vi "FL Sigmoid COA Single Side.vi"(0 "weight":dbl, 5 "Implication":T1 items=["Minimum", "Product"], 7 "x0":dbl=-5.0, 9 "x1":dbl=5.0, 11 "A":dbl=1.0) -> (4 "xlh":dbl, 6 "area":dbl, 8 "coa_x":dbl, 10 "x_l":dbl, 15 "x_r":dbl)   [LabVIEW 2017, in "NI_Fuzzy_Logic_API.lvlib"]
uses:
  <vilib>/addons/Fuzzy Logic/NI_Fuzzy_Logic_API.lvlib
  <vilib>/addons/Fuzzy Logic/TypeDefs/FL Consequent Implication.ctl
  <vilib>/gmath/NI_Gmath.lvlib
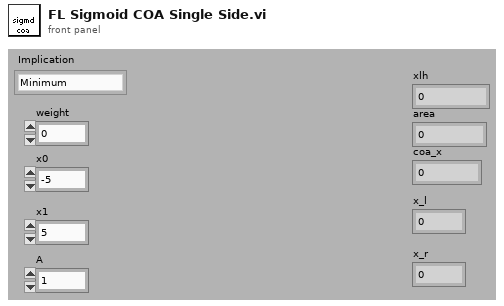
[diagram p1: front panel]
types:
  T1 = typedef "NI_Fuzzy_Logic_API.lvlib/FL Consequent Implication.ctl" = u16
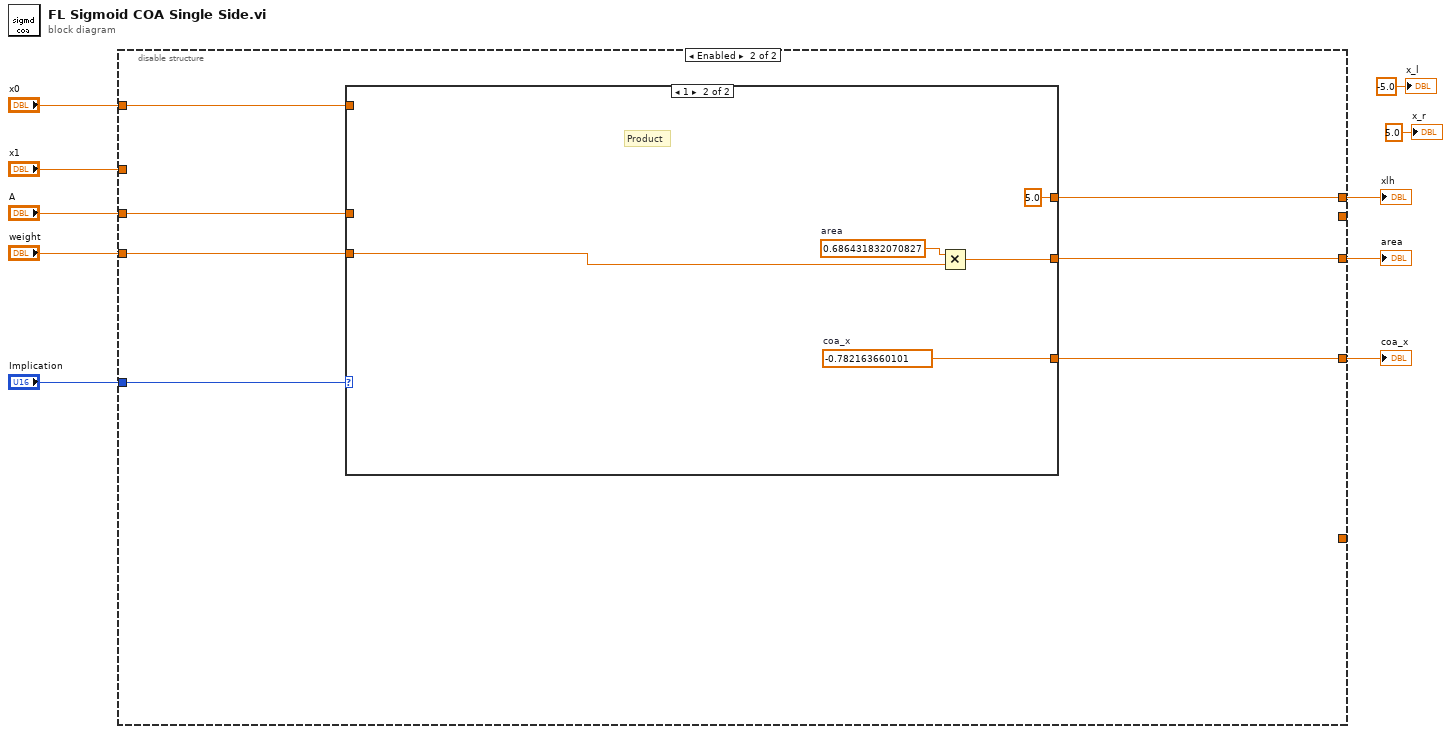
[diagram p0: block diagram]
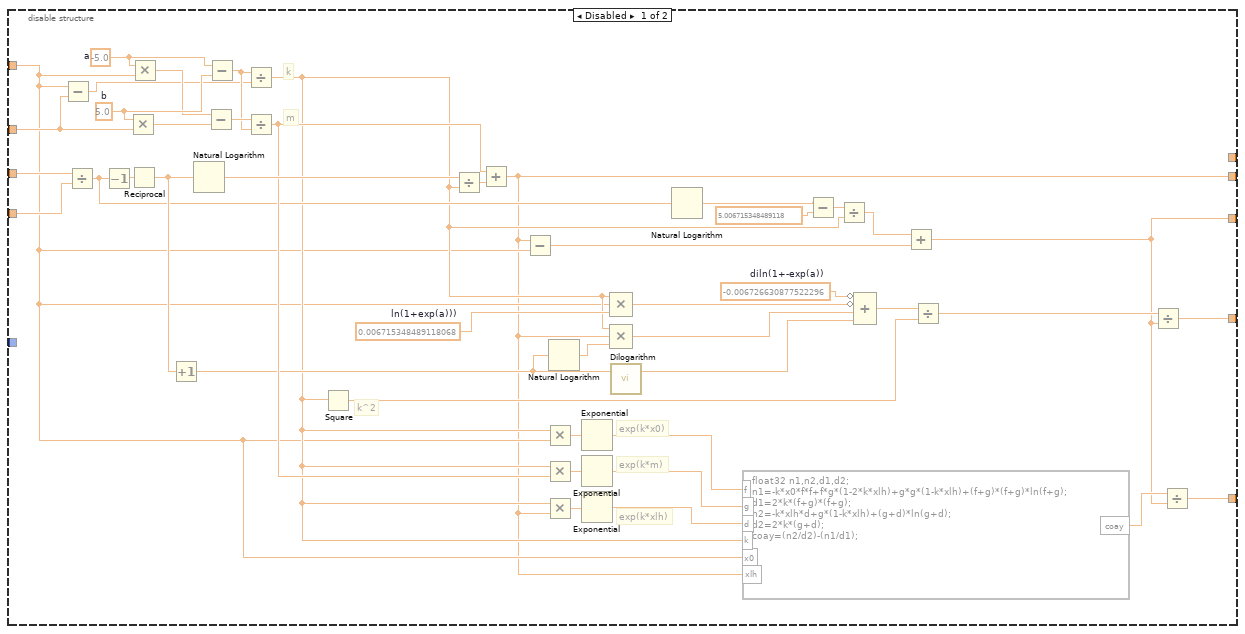
[diagram p2: hidden frame]
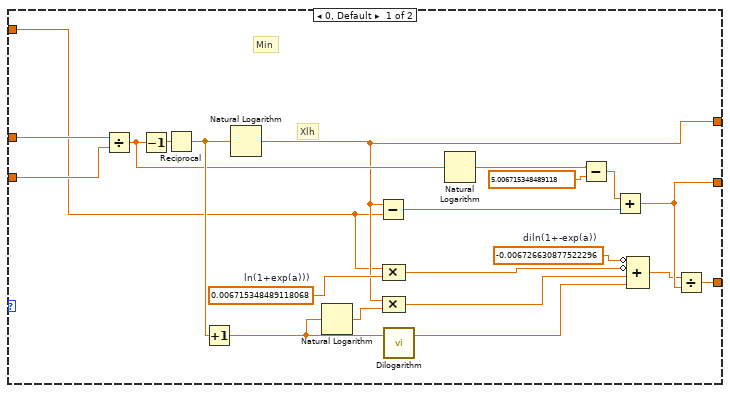
[diagram p3: hidden frame]
diagram:
  n1 = disable-structure shown="Enabled" {
    disable-tunnel: "x1" -> [w50 _]
    disable-tunnel: "A" -> [w43 w61]
    disable-tunnel: "weight" -> [w42 w60]
    disable-tunnel: [w22 w59] -> w7
    disable-tunnel: "x0" -> [w20 w56]
    disable-tunnel: [w13 _] -> _
    disable-tunnel: [w12 w58] -> w5
    disable-tunnel: [w11 _] -> _
    disable-tunnel: [_ w57] -> w4
    disable-tunnel: "Implication" -> [_ w55]
    frame Disabled {
      w30 = -0.006726630877522296  # diln(1+-exp(a))
      w32 = 0.006715348489118068  # ln(1+exp(a)))
      w54 = 5.0  # b
      w33 = -5.0  # a
      # "k^2"
      # "exp(k*xlh)"
      # "exp(k*x0)"
      # "exp(k*m)"
      # "k"
      # "m"
      n2 = Subtract(x=w20, y=w50) -> (x-y=w48:dbl)
      n3 = Divide(x=w43, y=w42) -> (x/y=w31:dbl)
      n4 = Decrement(x=w31) -> (x-1=w41:dbl)
      n5 = Multiply(x=w54, y=w50) -> (x*y=w52:dbl)
      n6 = Reciprocal(x=w41) -> (1/x=w34:dbl)
      n7 = Multiply(x=w33, y=w20) -> (x*y=w53:dbl)
      n8 = Increment(x=w34) -> (x+1=w29:dbl)
      n9 = Natural Logarithm(1:w34) -> (0:w40:dbl)
      n10 = Subtract(x=w53, y=w52) -> (x-y=w51:dbl)
      n11 = Subtract(x=w33, y=w54) -> (x-y=w49:dbl)
      n12 = Divide(x=w49, y=w48) -> (x/y=w21:dbl)
      n13 = Divide(x=w51, y=w49) -> (x/y=w38:dbl)
      n14 = Square(x=w21) -> (x^2=w28:dbl)
      n15 = Divide(x=w40, y=w21) -> (x/y=w39:dbl)
      n16 = Add(x=w38, y=w39) -> (x+y=w13:dbl)
      n17 = Subtract(x=w13, y=w20) -> (x-y=w36:dbl)
      n18 = Multiply(x=w21, y=w20) -> (x*y=w18:dbl)
      n19 = Multiply(x=w21, y=w38) -> (x*y=w37:dbl)
      n20 = Multiply(x=w21, y=w13) -> (x*y=w16:dbl)
      n21 = Natural Logarithm(1:w29) -> (0:w27:dbl)
      n22 = Exponential(1:w18) -> (0:w17:dbl)
      n23 = Exponential(1:w37) -> (0:w14:dbl)
      n24 = Exponential(1:w16) -> (0:w15:dbl)
      n25 = Compound Arithmetic op=MULTIPLY(w21, w20, w32) -> (w47:dbl)
      n26 = Compound Arithmetic op=MULTIPLY(w21, w13, w27) -> (w46:dbl)
      n27 = call <vilib>:"Dilogarithm.vi"("x"=w29) -> ("diln(x)"=w45:dbl)  [unwired: 2 out]
      n28 = Natural Logarithm(1:w31) -> (0:w26:dbl)
      n29 = formula code="float32 n1,n2,d1,d2;\nn1=-k*x0*f*f+f*g*(1-2*k*xlh)+g*g*(1-k*xlh)+(f+g)*(f+g)*ln(f+g);\nd1=2*k*(f+g)*(f+g);\nn2=-k*xlh*d+g*(1-k*xlh)+(g+d)*ln(g+d);\nd2=2*k*(g+d);\ncoay=(n2/d2)-(n1/d1);"("d"=w15, "f"=w17, "g"=w14, "x0"=w20, "k"=w21, "xlh"=w13) -> ("coay"=w19:dbl)
      n30 = Subtract(x=w26, y=5.006715348489118 ("ln(x+1)")) -> (x-y=w24:dbl)
      n31 = Divide(x=w24, y=w21) -> (x/y=w35:dbl)
      n32 = Compound Arithmetic op=ADD(invert w30, invert w47, w46, w45) -> (w44:dbl)
      n33 = Add(x=w35, y=w36) -> (x+y=w12:dbl)
      n34 = Divide(x=w44, y=w28) -> (x/y=w23:dbl)
      n35 = Divide(x=w23, y=w12) -> (x/y=w22:dbl)
      n36 = Divide(x=w19, y=w12) -> (x/y=w11:dbl)
    }
    frame Enabled {
      n37 = case shown="1" w55 {
        tunnel: w61 -> [w79 _]
        tunnel: w60 -> [w78 w84]
        tunnel: [w67 w83] -> w59
        tunnel: [w66 w85] -> w58
        tunnel: [w63 5.0] -> w57
        tunnel: w56 -> [w62 _]
        frame 0, Default {
          w72 = -0.006726630877522296  # diln(1+-exp(a))
          w74 = 0.006715348489118068  # ln(1+exp(a)))
          # "Min"
          # "Xlh"
          n38 = Divide(x=w79, y=w78) -> (x/y=w73:dbl)
          n39 = Decrement(x=w73) -> (x-1=w77:dbl)
          n40 = Reciprocal(x=w77) -> (1/x=w75:dbl)
          n41 = Increment(x=w75) -> (x+1=w71:dbl)
          n42 = Natural Logarithm(1:w75) -> (0:w63:dbl)
          n43 = Natural Logarithm(1:w71) -> (0:w70:dbl)
          n44 = Subtract(x=w63, y=w62) -> (x-y=w76:dbl)
          n45 = Compound Arithmetic op=MULTIPLY(w62, w74) -> (w82:dbl)
          n46 = Compound Arithmetic op=MULTIPLY(w63, w70) -> (w81:dbl)
          n47 = call <vilib>:"Dilogarithm.vi"("x"=w71) -> ("diln(x)"=w80:dbl)  [unwired: 2 out]
          n48 = Natural Logarithm(1:w73) -> (0:w69:dbl)
          n49 = Subtract(x=w69, y=5.006715348489118 ("ln(x+1)")) -> (x-y=w65:dbl)
          n50 = Add(x=w65, y=w76) -> (x+y=w66:dbl)
          n51 = Compound Arithmetic op=ADD(invert w72, invert w82, w81, w80) -> (w64:dbl)
          n52 = Divide(x=w64, y=w66) -> (x/y=w67:dbl)
        }
        frame 1 {
          w83 = -0.782163660101  # coa_x
          w86 = 0.686431832070827  # area
          # "Product"
          n53 = Multiply(x=w86, y=w84) -> (x*y=w85:dbl)
        }
      }
    }
  }
  "area" <- w5
  "coa_x" <- w7
  "xlh" <- w4
  "x_l" <- -5.0 ("x_l")
  "x_r" <- 5.0 ("x_r")
